vi "Example4.vi"() -> ()   [LabVIEW 2020, in "LcPictureBox.lvclass"]
uses:
  LcPictureBox.lvclass
  System.Windows.Forms
  SmoothingMode.ctl
panel:
  in  "PictureBox 1":refnum<k24>(container)
  out "error out":errorcluster
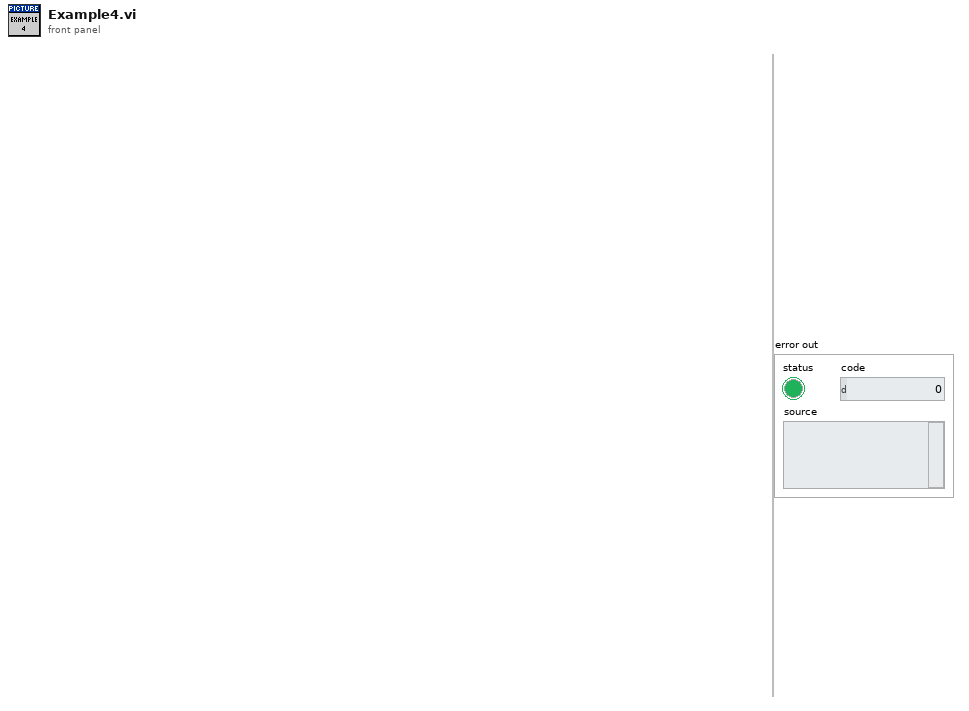
[diagram p1: front panel]
types:
  T1 = cluster{"horizontal":enum16{"Left", "Center", "Right"}, "vertical":enum16{"Top", "Center", "Bottom"}}
  T2 = typedef "LcPictureBox.lvclass/SmoothingMode.ctl" = enum16{"None", "HighSpeed", "HighQuality", "AntiAlias"}
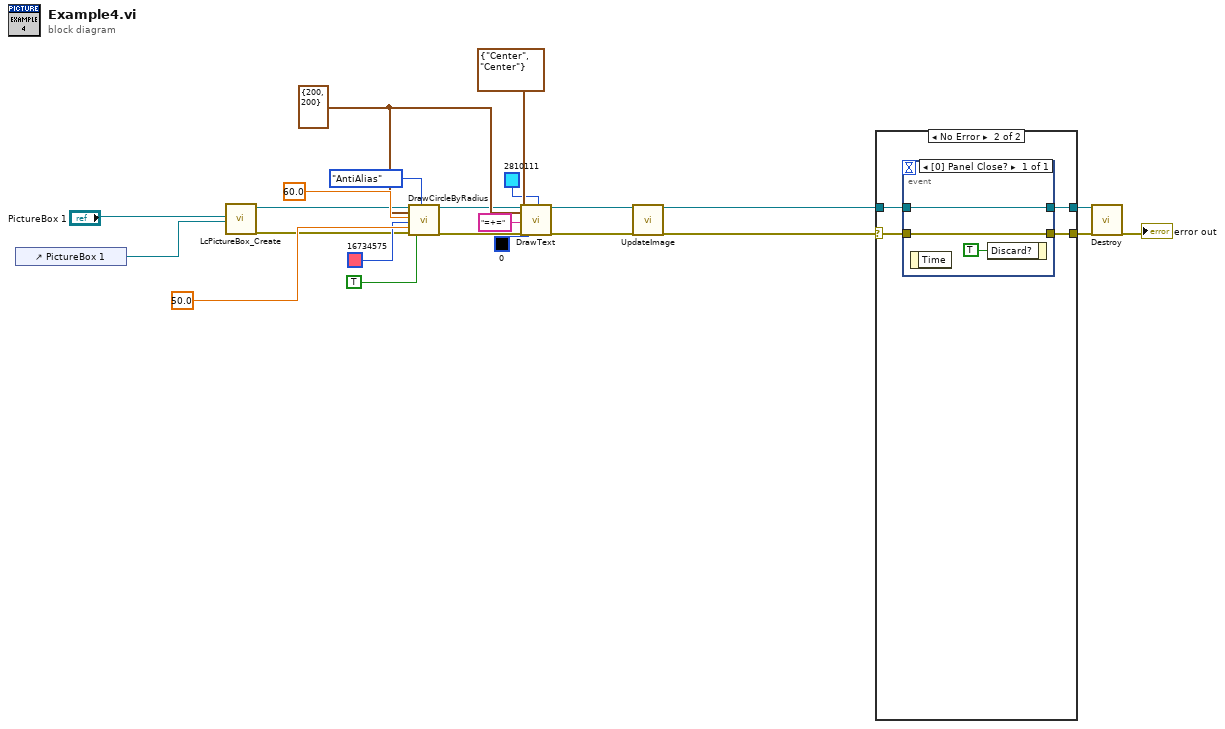
[diagram p0: block diagram]
diagram:
  w8 = cluster{"x":i32, "y":i32} {"x"=200, "y"=200} ("Point")
  n1 = control-ref of="PictureBox 1"() -> (w2:refnum<vi>)
  n2 = call "LcPictureBox_Create.vi"("PictureBox"="PictureBox 1", "PictureBoxActiveXReference"=w2) -> ("reference out"=w14:refnum<class "LcPictureBox.lvclass">, "Error Out"=w13:errorcluster)  [unwired: 15 in, 1 out]
  n3 = call-dynamic "DrawCircleByRadius.vi"("reference in"=w14, "Center"=w8, "Radius"=sgl 60.0, "Color(Black)"=u32 16734575, "Alpha(100%)"=50.0, "Error In"=w13, "Fill(False)"=TRUE, "SmoothingMode(AntiAlias)"=SmoothingMode."AntiAlias" ("SmoothingMode")) -> ("reference out"=w1:refnum<class "LcPictureBox.lvclass">, "Error Out"=w12:errorcluster)  [unwired: 10 in]
  n4 = call-dynamic "DrawText.vi"("reference in"=w1, "Origin"=w8, "Alignment(Left,Top)"=T1 {"horizontal"=enum."Center", "vertical"=enum."Center"}, "Text"="=+=", "Error In"=w12, "Color(Black)"=u32 0, "BgColor(Transparent)"=u32 2810111) -> ("reference out"=w9:refnum<class "LcPictureBox.lvclass">, "Error Out"=w10:errorcluster)  [unwired: 11 in]
  n5 = call-dynamic "UpdateImage.vi"("reference in"=w9, "Error In"=w10) -> ("reference out"=w19:refnum<class "LcPictureBox.lvclass">, "Error Out"=w3:errorcluster)  [unwired: 14 in, 2 out]
  n6 = case shown="No Error" w3 {
    selector: w3 -> [w25 w26]
    tunnel: [w25 w29] -> w22
    tunnel: w19 -> [w24 w28]
    tunnel: [w24 w27] -> w21
    frame Error {
    }
    frame No Error {
      n7 = event shown="[0] Panel Close?" {
        selector: _ -> [_]
        dyn-events: _ -> [_]
        timeout: _ -> [_]
        tunnel: w26 -> [w31]
        tunnel: [w31] -> w29
        tunnel: w28 -> [w30]
        tunnel: [w30] -> w27
        event Panel Close? {
          n8 = event-data() -> ()  [unwired: 1 in, 1 out]
          n9 = event-data("Discard?"=TRUE) -> ()  [unwired: 1 in, 1 out]
        }
      }
    }
  }
  n10 = call-dynamic "Destroy.vi"("reference in"=w21, "Error In"=w22) -> ("Error Out"=→"error out":errorcluster)  [unwired: 16 in, 1 out]
